vi "Path String to Path(Relative Path).vi"(1 "String":string) -> (0 "Path":path)   [LabVIEW 2017]
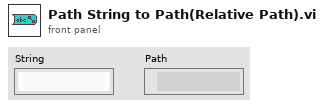
[diagram p1: front panel]
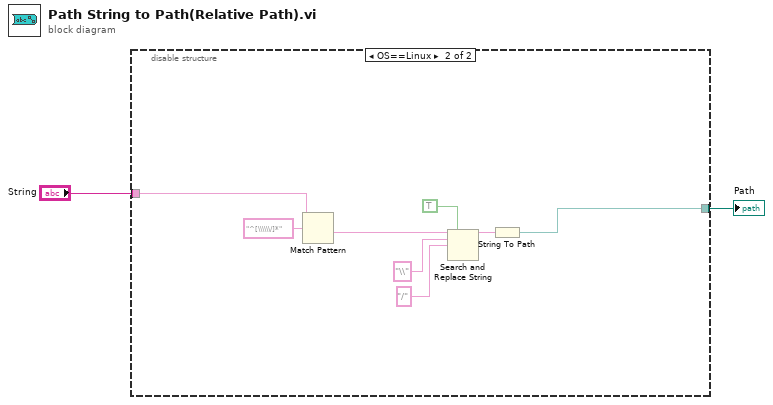
[diagram p0: block diagram]
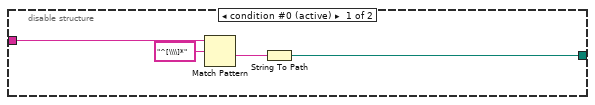
[diagram p2: hidden frame]
diagram:
  n1 = disable-structure shown="OS==Linux" {
    disable-tunnel: [w5 w7] -> w2
    disable-tunnel: "String" -> [w4 w13]
    frame condition #0 (active) {
      n2 = Match Pattern(string=w4, regular expression="^[\\\\]*") -> (after substring=w6:string)  [unwired: 1 in, 3 out]
      n3 = String To Path(string=w6) -> (path=w5:path)
    }
    frame condition #1 {
      n4 = Match Pattern(string=w13, regular expression="^[\\\\\\/]*") -> (after substring=w12:string)  [unwired: 1 in, 3 out]
      n5 = Search and Replace String(replace all?=TRUE ("replace all? (F)"), input string=w12, search string="\\" ("regular expression"), replace string="/" ("regular expression")) -> (result string=w8:string)  [unwired: 4 in, 3 out]
      n6 = String To Path(string=w8) -> (path=w7:path)
    }
  }
  "Path" <- w2
